vi "Calculate New Analysis Start And End Angle.vi"(8 "Right Wing?":bool, 9 "End Angle":fxp<+/-,17,2>, 10 "Start Angle":fxp<+/-,17,2>, 11 "Sector":u8) -> (2 "Start Angle Out":fxp<+/-,17,2>, 3 "End Angle Out":fxp<+/-,17,2>)   [LabVIEW 2013]
uses:
  <vilib>/rvi/Analysis/common/FxpNativeNode/niFpgaFxpNative.xnode
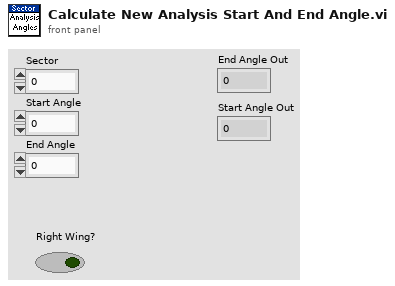
[diagram p1: front panel]
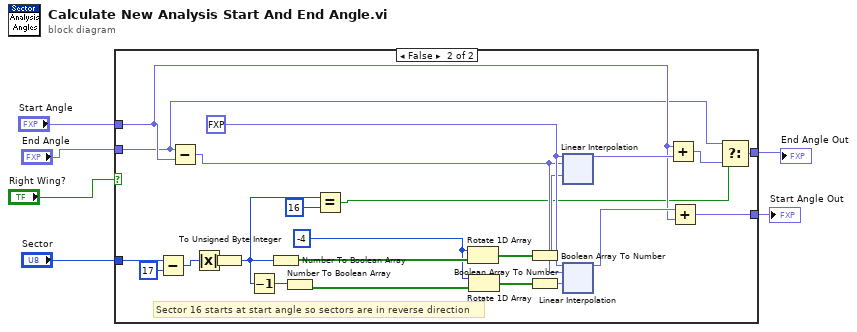
[diagram p0: block diagram]
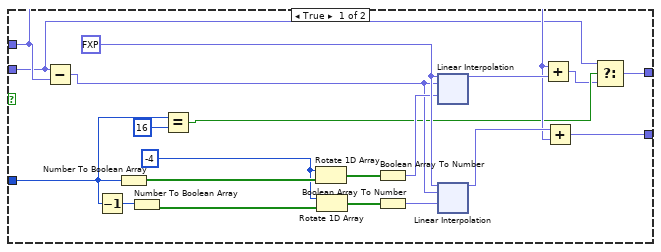
[diagram p2: hidden frame]
diagram:
  n1 = case shown="False" "Right Wing?" {
    tunnel: "Start Angle" -> [w14 w60]
    tunnel: [w13 w59] -> w5
    tunnel: "Sector" -> [w12 w58]
    tunnel: [w8 w54] -> w3
    tunnel: "End Angle" -> [w7 w53]
    frame True {
      w22 = -4 ("n")
      w18 = fxp<+/-,17,2> 0.0 ("Start Angle")
      n2 = Subtract(x=w7, y=w14) -> (x-y=w16:fxp<+/-,18,2>)
      n3 = Decrement(x=w12) -> (x-1=w23:u8)
      n4 = Number To Boolean Array(number=w12) -> (Boolean array=w25:bool[])
      n5 = Number To Boolean Array(number=w23) -> (Boolean array=w21:bool[])
      n6 = Equal?(x=w12, y=u8 16) -> (x = y?=w10:bool)
      n7 = Rotate 1D Array(1:w25, 2:w22) -> (0:w24:bool[])
      n8 = Rotate 1D Array(1:w21, 2:w22) -> (0:w20:bool[])
      n9 = Boolean Array To Number(Boolean array=w24) -> (number=w17:fxp<+,8,0>)
      n10 = Boolean Array To Number(Boolean array=w20) -> (number=w19:fxp<+,8,0>)
      n11 = xnode ("Linear Interpolation")("y0"=w18, "y1"=w16, "x"=w17) -> ("y"=w26:fxp<+/-,17,2>)
      n12 = xnode ("Linear Interpolation")("y0"=w18, "y1"=w16, "x"=w19) -> ("y"=w15:fxp<+/-,17,2>)
      n13 = Add(x=w14, y=w26) -> (x+y=w9:fxp<+/-,17,2>)
      n14 = Add(x=w15, y=w14) -> (x+y=w13:fxp<+/-,17,2>)
      n15 = Select(t=w7, s=w10, f=w9) -> (s? t:f=w8:fxp<+/-,17,2>)
    }
    frame False {
      w68 = -4 ("n")
      w64 = fxp<+/-,17,2> 0.0 ("Start Angle")
      # "Sector 16 starts at start angle so sectors are in reverse direction"
      n16 = Subtract(x=w58, y=i16 17) -> (x-y=w50:i16)
      n17 = Subtract(x=w53, y=w60) -> (x-y=w62:fxp<+/-,18,2>)
      n18 = Absolute Value(x=w50) -> (abs(x)=w51:i16)
      n19 = To Unsigned Byte Integer(number=w51) -> (unsigned 8bit integer=w49:u8)
      n20 = Decrement(x=w49) -> (x-1=w69:u8)
      n21 = Number To Boolean Array(number=w49) -> (Boolean array=w71:bool[])
      n22 = Number To Boolean Array(number=w69) -> (Boolean array=w67:bool[])
      n23 = Equal?(x=w49, y=u8 16) -> (x = y?=w56:bool)
      n24 = Rotate 1D Array(1:w71, 2:w68) -> (0:w70:bool[])
      n25 = Rotate 1D Array(1:w67, 2:w68) -> (0:w66:bool[])
      n26 = Boolean Array To Number(Boolean array=w70) -> (number=w63:fxp<+,8,0>)
      n27 = Boolean Array To Number(Boolean array=w66) -> (number=w65:fxp<+,8,0>)
      n28 = xnode ("Linear Interpolation")("y0"=w64, "y1"=w62, "x"=w63) -> ("y"=w72:fxp<+/-,17,2>)
      n29 = xnode ("Linear Interpolation")("y0"=w64, "y1"=w62, "x"=w65) -> ("y"=w61:fxp<+/-,17,2>)
      n30 = Add(x=w60, y=w72) -> (x+y=w55:fxp<+/-,17,2>)
      n31 = Add(x=w61, y=w60) -> (x+y=w59:fxp<+/-,17,2>)
      n32 = Select(t=w53, s=w56, f=w55) -> (s? t:f=w54:fxp<+/-,17,2>)
    }
  }
  "End Angle Out" <- w3
  "Start Angle Out" <- w5
